vi "refresh list.vi"(4 "Board Col":i32=2, 8 "错误输入（无错误）":errorcluster, 9 "Index/ROW":i32, 10 "NEW element":string[](array[string]), 11 "listin":refnum<vi>) -> (0 "error out":errorcluster caption="错误输出", 1 "fail counts":i32, 2 "Pf":string)   [LabVIEW 2018]
uses:
  <vilib>/Utility/miscctls.llb/LVRowAndColumnTypeDef.ctl
panel:
  in  "TEST":i32(listbox)
  in  "list":i32(listbox)
  in  "data out":string[](array[string])=["VAT", "0.3", "OFF", "1", "0.30503", "0.29497", "999.999990", "NG", "1000.211990", "999.787990", "", "NG", "1000.201990", "1000.201990", "0.000000", "NG"]
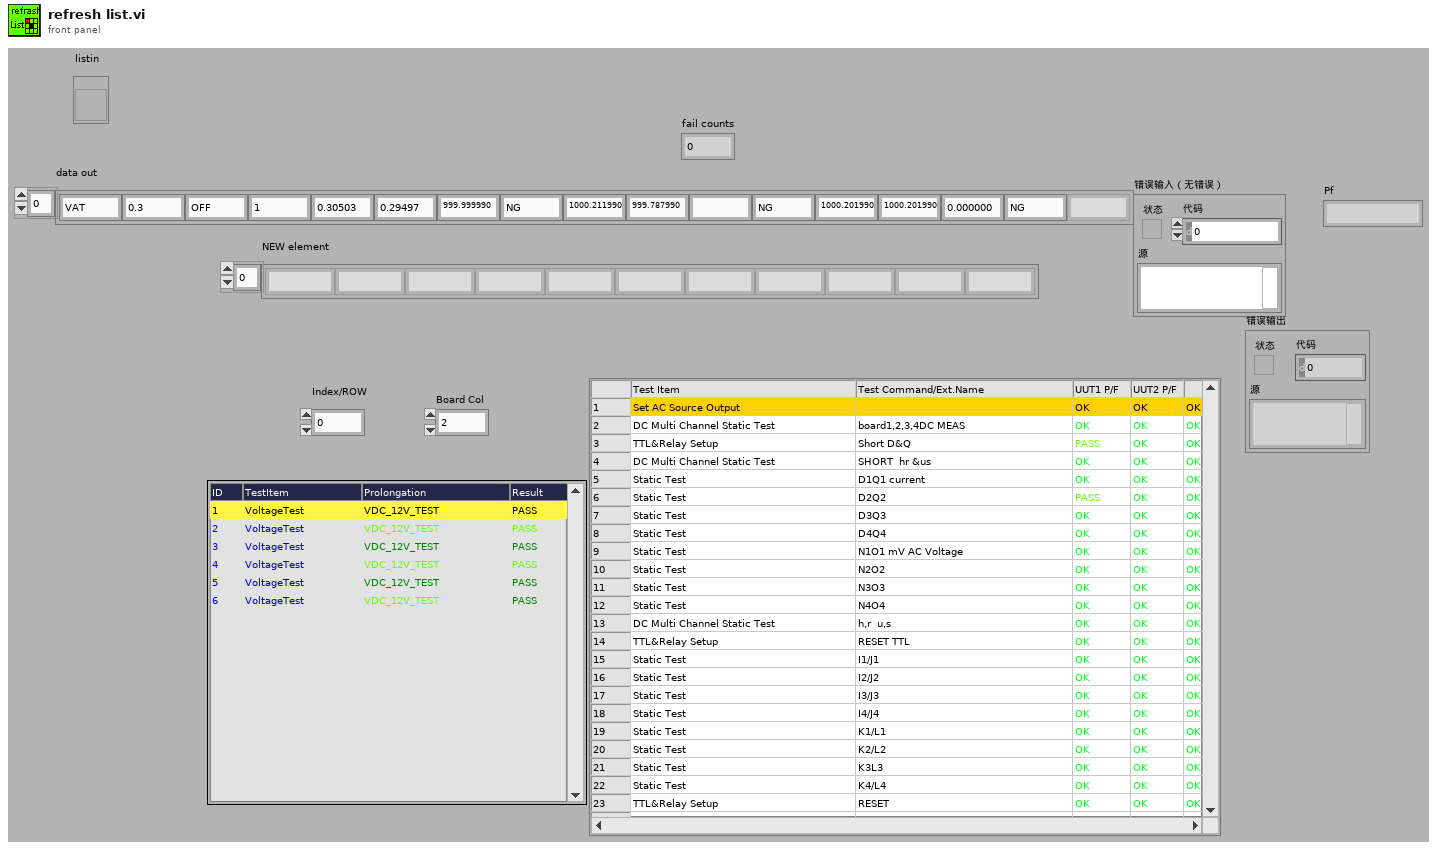
[diagram p1: front panel]
types:
  T1 = typedef "LVRowAndColumnTypeDef.ctl" = cluster{"Row":i32, "Column":i32}
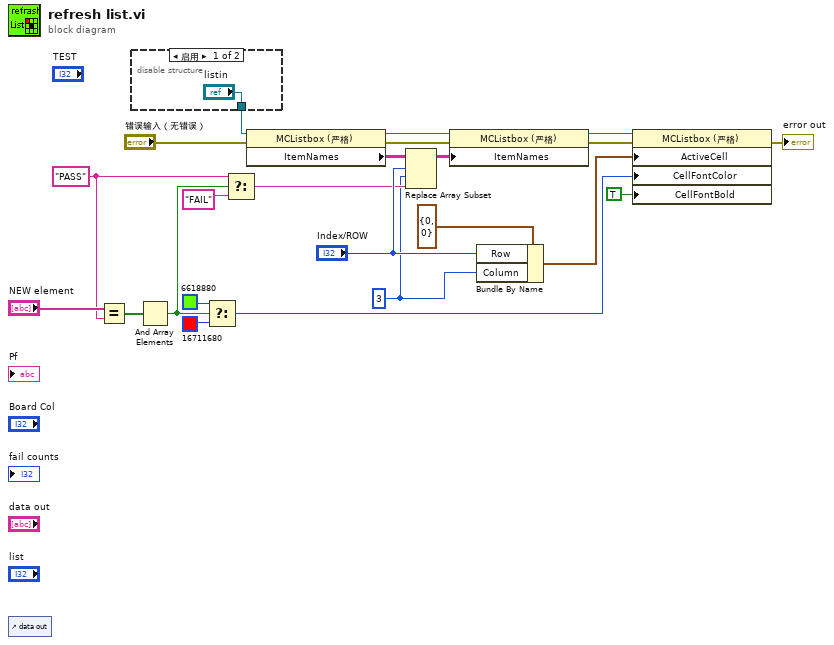
[diagram p0: block diagram]
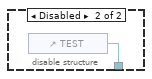
[diagram p2: hidden frame]
diagram:
  w1 = 3
  w13 = "PASS"
  n1 = control-ref of="data out"() -> ()  [unwired: 1 out]
  n2 = Equal?(x="NEW element", y=w13) -> (x = y?=w14:bool[])
  n3 = disable-structure shown="启用" {
    disable-tunnel: ["listin" w25] -> w19
    frame Enabled {
    }
    frame Disabled {
      n4 = control-ref of="TEST"() -> (w25:refnum<vi>)
    }
  }
  n5 = And Array Elements(Boolean array=w14) -> (logical AND=w4:bool)
  n6 = Select(t=u32 6618880, s=w4, f=u32 16711680) -> (s? t:f=w2:u32)
  n7 = Select(t=w13, s=w4, f="FAIL") -> (s? t:f=w11:string)
  n8 = property class="MCListbox (严格)"(reference=w19, error in="错误输入（无错误）") -> (reference out=w18:refnum<vi>, error out=w17:errorcluster, "ItemNames"=w15:string[][])
  n9 = Replace Array Subset ("替换数组子集")(array=w15, new element=w11, index (row)="Index/ROW", index (col)=w1) -> (w16:string[][])
  n10 = property class="MCListbox (严格)"(reference=w18, error in=w17, "ItemNames"=w16) -> (reference out=w8:refnum<vi>, error out=w7:errorcluster)
  n11 = Bundle By Name(cluster=T1 {"Row"=0, "Column"=0} ("活动单元格:活动单元格"), "Row"="Index/ROW", "Column"=w1) -> (w9:T1)
  n12 = property class="MCListbox (严格)"(reference=w8, error in=w7, "ActiveCell"=w9, "CellFontColor"=w2, "CellFontBold"=TRUE ("活动单元格:单元格字体:粗体")) -> (error out=→"error out":errorcluster)  [unwired: 1 out]
